vi "NetVarWrite_bool.vi"(8 "data in":bool, 11 "Refnum in":refnum<k21>) -> ()   [LabVIEW 2016]
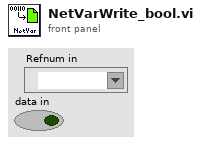
[diagram p1: front panel]
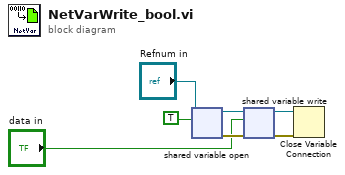
[diagram p0: block diagram]
diagram:
  n1 = shared-variable-open("Refnum in", TRUE) -> (w5:refnum<k21>, w4:errorcluster)  [unwired: 2 in]
  n2 = shared-variable-write(w5, w4, "data in") -> (w6:refnum<k21>, w3:errorcluster)
  n3 = Close Variable Connection(8:w3, 11:w6) -> ()  [unwired: 1 out]
